vi "DSF.Engine.Transceiver Thread.Get Cache.vi"(11 "Transceiver Thread in":refnum<class "DSF.Engine.Transceiver Thread.lvclass">) -> (2 "Cache":refnum<class "DSF.Engine.Memory.Cache.lvclass">, 3 "Transceiver Thread out":refnum<class "DSF.Engine.Transceiver Thread.lvclass">)   [LabVIEW 2017, in "DSF.Engine.lvlib" / "DSF.Engine.Transceiver Thread.lvclass"]
uses:
  DSF.Engine.Transceiver Thread.lvclass
  Cache/DSF.Engine.Memory.Cache.lvclass
  DSF.Engine.Transceiver Thread.lvclass/DSF.Engine.Transceiver Thread.ctl
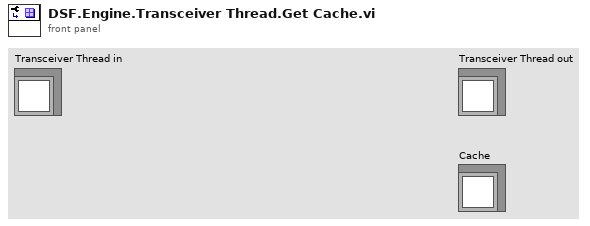
[diagram p1: front panel]
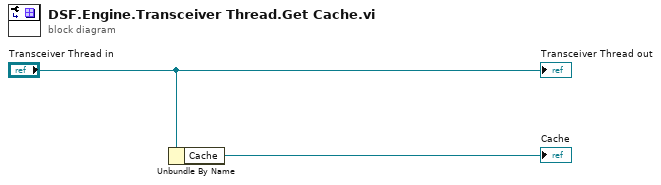
[diagram p0: block diagram]
diagram:
  n1 = Unbundle By Name("Transceiver Thread in") -> ("Cache"=→"Cache":refnum<class "DSF.Engine.Memory.Cache.lvclass">)
  "Transceiver Thread out" <- "Transceiver Thread in"
